vi "checkreg.vi"(0 "error in (no error)":errorcluster) -> (1 "Boolean":bool, 2 "error out 2":errorcluster caption="error out")   [LabVIEW 2014]
uses:
  <vilib>/registry/registry.llb/Registry RtKey.ctl
  <vilib>/registry/registry.llb/Registry SAM.ctl
  <vilib>/registry/registry.llb/Read Registry Value Simple STR.vi
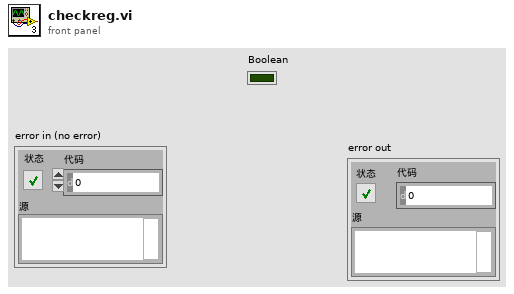
[diagram p1: front panel]
types:
  T1 = typedef "Registry SAM.ctl" = enum32{"KEY_QUERY_VALUE", "KEY_SET_VALUE", "KEY_CREATE_SUB_KEY", "KEY_ENUMERATE_SUB_KEYS", "KEY_NOTIFY", "KEY_CREATE_LINK", "KEY_READ", "KEY_WRITE", "KEY_ALL_ACCESS", "KEY_READ | KEY_WRITE"}
  T2 = typedef "Registry RtKey.ctl" = enum32{"HKEY_CLASSES_ROOT", "HKEY_CURRENT_USER", "HKEY_LOCAL_MACHINE", "HKEY_USERS", "HKEY_PERFORMANCE_DATA", "HKEY_CURRENT_CONFIG", "HKEY_DYN_DATA"}
  T3 = typedef "Registry refnum.ctl" = refnum<k1>
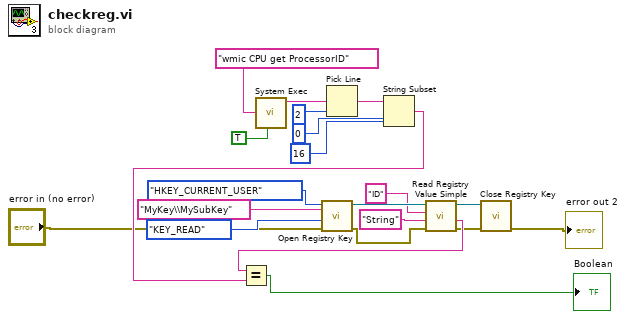
[diagram p0: block diagram]
diagram:
  n1 = call <vilib>:"System Exec.vi"("run minimized? (F)"=TRUE, "command line"="wmic CPU get ProcessorID") -> ("standard output"=w8:string)  [unwired: 6 in, 3 out]
  n2 = call <vilib>:"Open Registry Key.vi"("error in (no error)"="error in (no error)", "security access mask (KEY_READ | KEY_WRITE)"=Registry_SAM."KEY_READ", "subkey"="MyKey\\MySubKey", "root key (HKEY_LOCAL_MACHINE)"=Registry_RtKey."HKEY_CURRENT_USER") -> ("error out"=w13:errorcluster, "refnum out"=w18:T3)  [unwired: 6 in]
  n3 = Pick Line(multi-line string=w8, line index=2) -> (output string=w10:string)  [unwired: 1 in]
  n4 = String Subset(string=w10, offset (0)=0 ("偏移量(0)"), length (rest)=16 ("长度（剩余）")) -> (substring=w5:string)
  n5 = call-poly <vilib>:"Read Registry Value Simple.vi"("error in (no error)"=w13, "default data"="String", "value"="ID", "refnum"=w18) -> ("error out"=w14:errorcluster, "String/Binary data"=w15:string, "refnum out"=w17:T3)  [unwired: 2 in, 1 out]
  n6 = Equal?(x=w15, y=w5) -> (x = y?=→"Boolean":bool)
  n7 = call <vilib>:"Close Registry Key.vi"("error in (no error)"=w14, "refnum"=w17) -> ("error out"=→"error out 2":errorcluster)  [unwired: 5 in]
